vi "add 1.vi"(0 "Numeric 2":dbl, 3 "Numeric":dbl) -> (10 "Numeric 3":dbl)   [LabVIEW 2025]
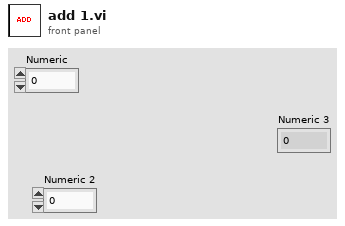
[diagram p1: front panel]
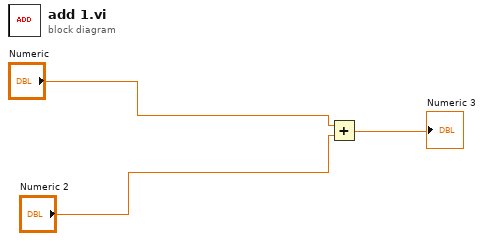
[diagram p0: block diagram]
diagram:
  n1 = Add(x="Numeric", y="Numeric 2") -> (x+y=→"Numeric 3":dbl)
